vi "test sort channels.vi"() -> (0 "no err":errorcluster, 3 "lookup ok":bool)   [LabVIEW 2013, in "TBM Tests.lvlib"]
uses:
  TBM Tests.lvlib
  channel/TBM channel.lvclass
  <vilib>/NI/Tag Bus/dictionary/data dictionary.lvclass
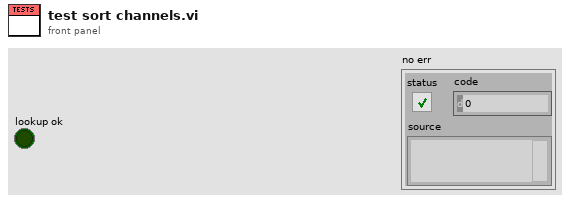
[diagram p1: front panel]
types:
  T1 = typedef "TBM channel.lvclass/channel classification.ctl" = enum16{"input data", "output data", "processing parameter", "processing result"}
  T2 = typedef "tag bus.lvlib/tag descriptor.lvclass/Data Type.ctl" = enum16{"Double", "Single", "I64", "I32", "I16", "I8", "U64", "U32", "U16", "U8", "Boolean", "String", "Array of Double", "Array of Single", "Array of I64", "Array of I32", "Array of I16", "Array of I8", "Array of U64", "Array of U32", "Array of U16", "Array of U8", "Array of Boolean", "Array of String"}
  T3 = typedef "TBM channel.lvclass/data tables.ctl" = cluster{"input data":T4, "processing parameter":T4, "processing result":T4, "output data":T4}
  T4 = typedef "tag bus.lvlib/dictionary table pair.ctl" = cluster{"data dictionary":refnum<class "data dictionary.lvclass">, "data table":T5}
  T5 = typedef "tag bus.lvlib/data table.lvlib/data table.ctl" = cluster{"Double":dbl[], "Single":sgl[], "I64":i64[], "I32":i32[], "I16":i16[], "I8":i8[], "U64":u64[], "U32":u32[], "U16":u16[], "U8":u8[], "Boolean":bool[], "String":string[], "Array of Double":cluster{"DBL Array":dbl[]}[], "Array of Single":cluster{"SGL Array":sgl[]}[], "Array of I64":cluster{"I64 Array":i64[]}[], "Array of I32":cluster{"I32 Array":i32[]}[], "Array of I16":cluster{"I16 Array":i16[]}[], "Array of I8":cluster{"I8 Array":i8[]}[], "Array of U64":cluster{"U64 Array":u64[]}[], "Array of U32":cluster{"U32 Array":u32[]}[], "Array of U16":cluster{"U16 Array":u16[]}[], "Array of U8":cluster{"U8 Array":u8[]}[], "Array of Boolean":cluster{"Boolean Array":bool[]}[], "Array of String":cluster{"String Array":string[]}[]}
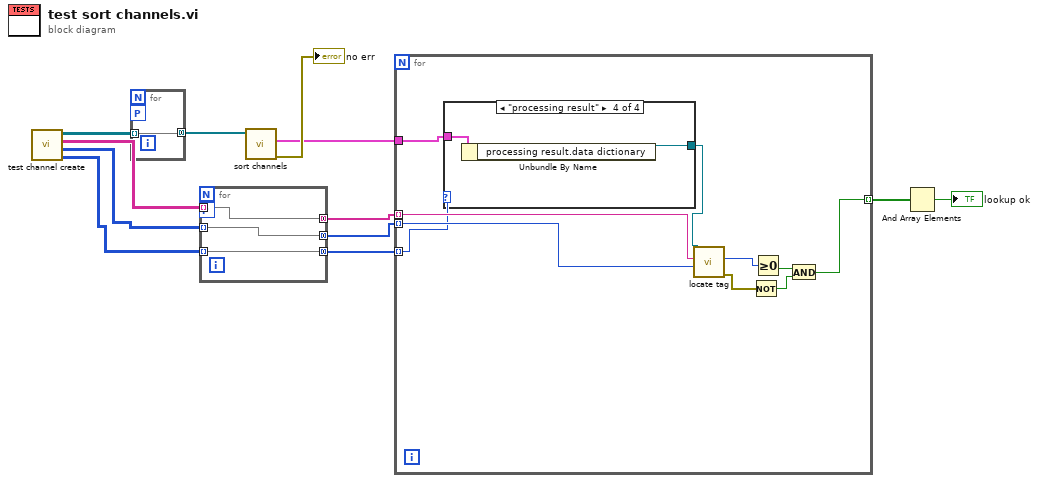
[diagram p0: block diagram]
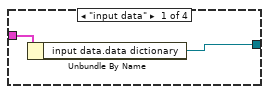
[diagram p2: hidden frame]
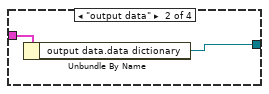
[diagram p3: hidden frame]
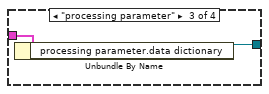
[diagram p4: hidden frame]
diagram:
  n1 = call "test channel create.vi"() -> ("dirs"=w1:T1[][], "types"=w3:T2[][], "names"=w5:string[][], "chans"=w12:refnum<class "TBM channel.lvclass">[][])  [unwired: 5 in, 3 out]
  n2 = for {
    tunnel: w12 -> [w13] mode=indexing
    tunnel: [w13] -> w10 mode=concatenating
    workers-P: _ -> [_]
  }
  n3 = for {
    tunnel: [w16] -> w6 mode=concatenating
    tunnel: w5 -> [w16] mode=indexing
    tunnel: [w15] -> w4 mode=concatenating
    tunnel: w3 -> [w15] mode=indexing
    tunnel: [w14] -> w2 mode=concatenating
    tunnel: w1 -> [w14] mode=indexing
    workers-P: _ -> [_]
  }
  n4 = call "sort channels.vi"("channels in"=w10) -> ("error out"=→"no err":errorcluster, "data allocations"=w8:T3)  [unwired: 8 in, 1 out]
  n5 = for {
    tunnel: w6 -> [w25] mode=indexing
    tunnel: w4 -> [w24] mode=indexing
    tunnel: w8 -> [w26]
    tunnel: [w23] -> w7 mode=indexing
    tunnel: w2 -> [w17] mode=indexing
    n6 = case shown="\"processing result\"" w17 {
      tunnel: w26 -> [w28 w30 w32 w34]
      tunnel: [w27 w29 w31 w33] -> w18
      frame "input data" {
        n7 = Unbundle By Name(w28) -> ("input data.data dictionary"=w27:refnum<class "data dictionary.lvclass">)
      }
      frame "output data" {
        n8 = Unbundle By Name(w30) -> ("output data.data dictionary"=w29:refnum<class "data dictionary.lvclass">)
      }
      frame "processing parameter" {
        n9 = Unbundle By Name(w32) -> ("processing parameter.data dictionary"=w31:refnum<class "data dictionary.lvclass">)
      }
      frame "processing result" {
        n10 = Unbundle By Name(w34) -> ("processing result.data dictionary"=w33:refnum<class "data dictionary.lvclass">)
      }
    }
    n11 = call <vilib>:"locate tag.vi"("data type"=w24, "name"=w25, "data dictionary in"=w18) -> ("error out"=w21:errorcluster, "index"=w22:i32)  [unwired: 6 in, 1 out]
    n12 = Not(x=w21) -> (.not. x?=w19:bool)
    n13 = Greater Or Equal To 0?(x=w22) -> (x >= 0?=w20:bool)
    n14 = And(x=w20, y=w19) -> (x .and. y?=w23:bool)
  }
  n15 = And Array Elements(Boolean array=w7) -> (logical AND=→"lookup ok":bool)
